vi "Test A3200 Axis.vi"() -> ()   [LabVIEW 2026]
uses:
  <instrlib>/A3200/Motion/AbortSingle.vi
  <instrlib>/A3200/Motion/FreerunSingle.vi
  <instrlib>/A3200/Motion/HomeSingle.vi
panel:
  out "NewVal":enum32{"X", "Y", "Z"}(ring)
  in  "Axis Control":enum32{"X", "Y", "Z"}(radio)
  in  "HOME":bool
  in  "SPEED I AM SPEED":dbl
  in  "GO LEFT":bool
  in  "Stop":bool
  in  "ACKNOWLEDGE ALL":bool
  in  "GO RIGHT":bool
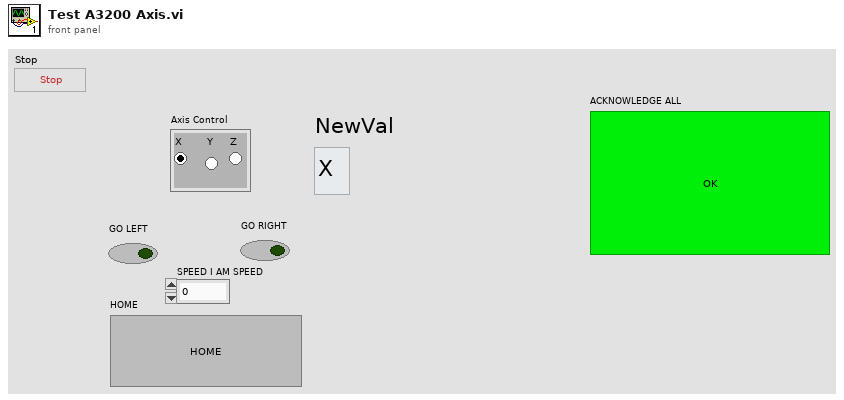
[diagram p1: front panel]
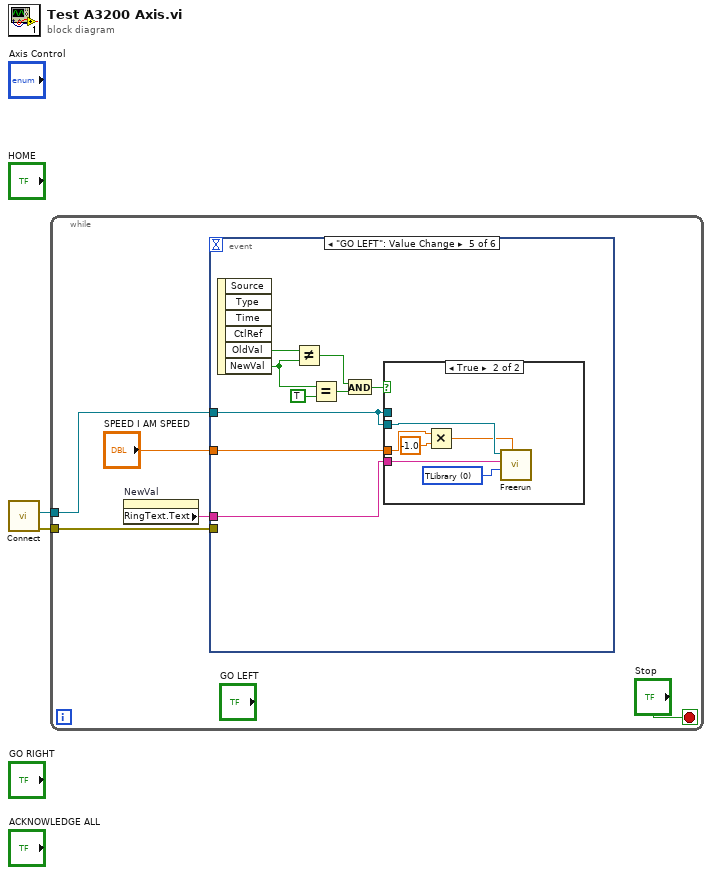
[diagram p0: block diagram]
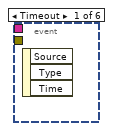
[diagram p2: hidden frame]
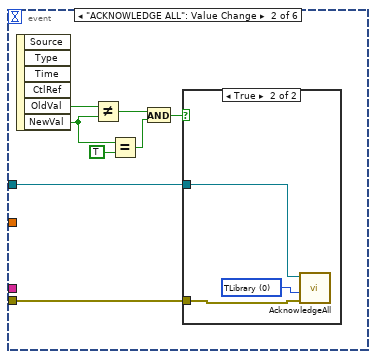
[diagram p3: hidden frame]
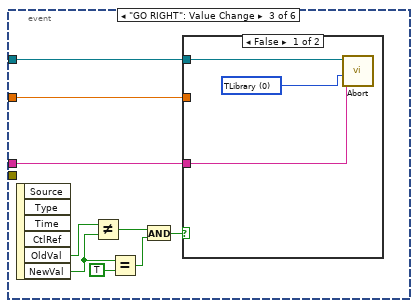
[diagram p5: hidden frame]
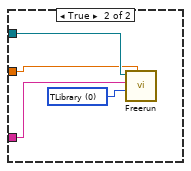
[diagram p6: hidden frame]
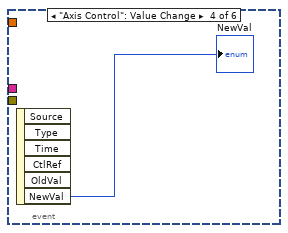
[diagram p7: hidden frame]
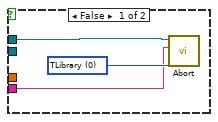
[diagram p8: hidden frame]
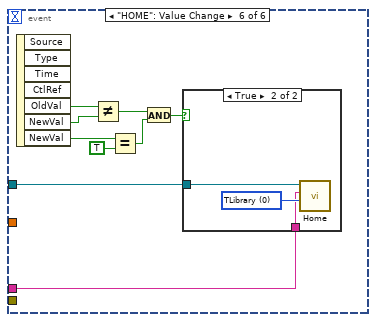
[diagram p9: hidden frame]
diagram:
  n1 = call <instrlib>:"Connect.vi"() -> ("error out"=w1:errorcluster, "controller"=w2:refnum<k24>)  [unwired: 10 in]
  n2 = while {
    tunnel: w2 -> [w7]
    tunnel: w1 -> [w6]
    stop <- "Stop" stop-if-true
    n3 = property on="NewVal" class="Enum (strict)"() -> ("RingText.Text"=w3:string)  [unwired: 2 in, 2 out]
    n4 = event shown="[4] \"GO LEFT\": Value Change" {
      selector: _ -> [_ _ _ _ _ _]
      dyn-events: _ -> [_ _ _ _ _ _]
      timeout: _ -> [_ _ _ _ _ _]
      tunnel: w7 -> [_ w15 w21 _ w38 w56]
      tunnel: w6 -> [_ w14 _ _ _ _]
      tunnel: "SPEED I AM SPEED" -> [_ _ w20 _ w37 _]
      tunnel: w3 -> [_ _ w19 _ w36 w54]
      event Timeout {
        n5 = event-data() -> ()  [unwired: 1 in, 3 out]
      }
      event "ACKNOWLEDGE ALL": Value Change {
        n6 = event-data() -> ("OldVal"=w13:bool, "NewVal"=w10:bool)  [unwired: 1 in, 4 out]
        n7 = Not Equal?(x=w13, y=w10) -> (x != y?=w12:bool)
        n8 = Equal?(x=w10, y=TRUE) -> (x = y?=w11:bool)
        n9 = And(x=w12, y=w11) -> (x .and. y?=w8:bool)
        n10 = case shown="True" w8 {
          tunnel: w15 -> [_ w18]
          tunnel: w14 -> [_ w17]
          frame False {
          }
          frame True {
            w16 = 0 items=["TLibrary", "T01", "T02", "T03", "T04", "T05", "T06", "T07", "T08", "T09", "T10", "T11", "T12", "T13", "T14", "T15", "T16", "T17", "T18", "T19", "T20", "T21", "T22", "T23", "T24", "T25", "T26", "T27", "T28", "T29", "T30", "T31"] ("taskId")
            n11 = call <instrlib>:"AcknowledgeAll.vi"("error in (no error)"=w17, "taskId"=w16, "controller in"=w18) -> ()  [unwired: 7 in, 2 out]
          }
        }
      }
      event "GO RIGHT": Value Change {
        n12 = event-data() -> ("OldVal"=w23:bool, "NewVal"=w22:bool)  [unwired: 1 in, 4 out]
        n13 = Not Equal?(x=w23, y=w22) -> (x != y?=w27:bool)
        n14 = Equal?(x=w22, y=TRUE) -> (x = y?=w26:bool)
        n15 = And(x=w27, y=w26) -> (x .and. y?=w24:bool)
        n16 = case shown="False" w24 {
          tunnel: w21 -> [w30 w34]
          tunnel: w20 -> [_ w32]
          tunnel: w19 -> [w28 w31]
          frame False {
            w29 = 0 items=["TLibrary", "T01", "T02", "T03", "T04", "T05", "T06", "T07", "T08", "T09", "T10", "T11", "T12", "T13", "T14", "T15", "T16", "T17", "T18", "T19", "T20", "T21", "T22", "T23", "T24", "T25", "T26", "T27", "T28", "T29", "T30", "T31"] ("taskId")
            n17 = call-poly <instrlib>:"Abort.vi"("taskId"=w29, "axis name? (all)"=w28, "controller in"=w30) -> ()  [unwired: 7 in, 2 out]
          }
          frame True {
            w33 = 0 items=["TLibrary", "T01", "T02", "T03", "T04", "T05", "T06", "T07", "T08", "T09", "T10", "T11", "T12", "T13", "T14", "T15", "T16", "T17", "T18", "T19", "T20", "T21", "T22", "T23", "T24", "T25", "T26", "T27", "T28", "T29", "T30", "T31"] ("taskId")
            n18 = call-poly <instrlib>:"Freerun.vi"("speed"=w32, "taskId"=w33, "axis name"=w31, "controller in"=w34) -> ()  [unwired: 6 in, 2 out]
          }
        }
      }
      event "Axis Control": Value Change {
        n19 = event-data() -> ("NewVal"=→"NewVal":enum32{"X", "Y", "Z"})  [unwired: 1 in, 5 out]
      }
      event "GO LEFT": Value Change {
        n20 = event-data() -> ("OldVal"=w41:bool, "NewVal"=w40:bool)  [unwired: 1 in, 4 out]
        n21 = Not Equal?(x=w41, y=w40) -> (x != y?=w44:bool)
        n22 = Equal?(x=w40, y=TRUE) -> (x = y?=w43:bool)
        n23 = And(x=w44, y=w43) -> (x .and. y?=w39:bool)
        n24 = case shown="True" w39 {
          tunnel: w38 -> [_ w52]
          tunnel: w38 -> [w46 _]
          tunnel: w37 -> [_ w50]
          tunnel: w36 -> [w45 w48]
          frame False {
            w47 = 0 items=["TLibrary", "T01", "T02", "T03", "T04", "T05", "T06", "T07", "T08", "T09", "T10", "T11", "T12", "T13", "T14", "T15", "T16", "T17", "T18", "T19", "T20", "T21", "T22", "T23", "T24", "T25", "T26", "T27", "T28", "T29", "T30", "T31"] ("taskId")
            n25 = call-poly <instrlib>:"Abort.vi"("taskId"=w47, "axis name? (all)"=w45, "controller in"=w46) -> ()  [unwired: 7 in, 2 out]
          }
          frame True {
            w53 = 0 items=["TLibrary", "T01", "T02", "T03", "T04", "T05", "T06", "T07", "T08", "T09", "T10", "T11", "T12", "T13", "T14", "T15", "T16", "T17", "T18", "T19", "T20", "T21", "T22", "T23", "T24", "T25", "T26", "T27", "T28", "T29", "T30", "T31"] ("taskId")
            n26 = Multiply(x=w50, y=-1.0) -> (x*y=w49:dbl)
            n27 = call-poly <instrlib>:"Freerun.vi"("speed"=w49, "taskId"=w53, "axis name"=w48, "controller in"=w52) -> ()  [unwired: 6 in, 2 out]
          }
        }
      }
      event "HOME": Value Change {
        n28 = event-data() -> ("OldVal"=w62:bool, "NewVal"=w61:bool, "NewVal"=w60:bool)  [unwired: 1 in, 4 out]
        n29 = Not Equal?(x=w62, y=w61) -> (x != y?=w57:bool)
        n30 = Equal?(x=w60, y=TRUE) -> (x = y?=w58:bool)
        n31 = And(x=w57, y=w58) -> (x .and. y?=w55:bool)
        n32 = case shown="True" w55 {
          tunnel: w56 -> [_ w65]
          tunnel: w54 -> [_ w63]
          frame False {
          }
          frame True {
            w64 = 0 items=["TLibrary", "T01", "T02", "T03", "T04", "T05", "T06", "T07", "T08", "T09", "T10", "T11", "T12", "T13", "T14", "T15", "T16", "T17", "T18", "T19", "T20", "T21", "T22", "T23", "T24", "T25", "T26", "T27", "T28", "T29", "T30", "T31"] ("taskId")
            n33 = call-poly <instrlib>:"Home.vi"("taskId"=w64, "axis name"=w63, "controller in"=w65) -> ()  [unwired: 7 in, 2 out]
          }
        }
      }
    }
  }
